vi "Configure PPS.vi"(8 "error in":errorcluster, 11 "PPS Config In":T2={"PPS Operation"=enum."Close", "PowerSupply Instrument"=enum."LVPPS", "Configure"={"Voltage Level (0.0 V)"=0.0, "CURRent Limit (0.0 A)"=0.0, "OVP LEVEL (0V)"=0.0, "OCP LEVEL (0A)"=0.0, "Enable OVP (T: Enable)"=TRUE, "Enable OCP (T: Enable)"=TRUE, "Enable Output "=TRUE, "Delays OCP"=0.0, "Delays OVP"=0.0, "Mode(0:Voltage)"=0, "CURRent Level (0.0 A)"=0.0, "Voltage Limit (0.0 V)"=0.0}} {"Configure"."Voltage Limit (0.0 V)" format="%.2f"; "Configure"."Mode(0:Voltage)" items=["Voltage", "Current"]; "Configure"."OCP LEVEL (0A)" format="%.2f"; "Configure"."OVP LEVEL (0V)" format="%.2f"; "Configure"."Voltage Level (0.0 V)" format="%.2f"}) -> (0 "error out":errorcluster, 3 "PPS Out":T1 {"Actual Current Limit (A)" format="%.2f"; "Actual Voltage Level (V)" format="%.2f"})   [LabVIEW 2023, in "GUI.lvlib" / "Diagnostic.lvlib"]
uses:
  Diagnostic.lvlib
  Control/PPS Configure UI.ctl
  HardwareAbstractionLayer_LVOOP/PowerSupply/Control/PPS Configure Data.ctl
  Control/PPS Out Data UI.ctl
  HardwareAbstractionLayer_LVOOP/PowerSupply/IT-M6018C/IT-M6018C.lvclass
  HardwareAbstractionLayer_LVOOP/PowerSupply/IT-M3904D/IT-M3904D.lvclass
  HardwareAbstractionLayer_LVOOP/PowerSupply/PowerSupply.lvclass
  HardwareAbstractionLayer_LVOOP/Database/Database.lvclass
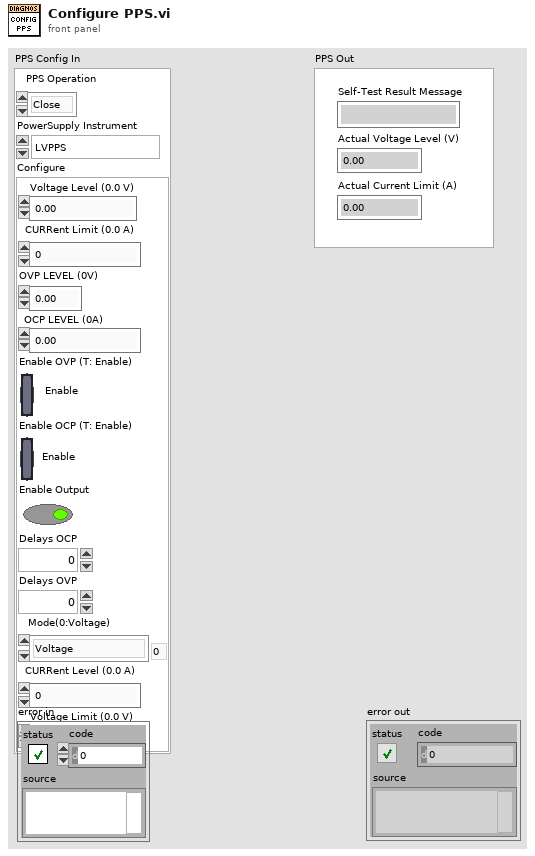
[diagram p1: front panel]
types:
  T1 = typedef "GUI.lvlib/Diagnostic.lvlib/PPS Out Data UI.ctl" = cluster{"Self-Test Result Message":string, "Actual Voltage Level (V)":dbl, "Actual Current Limit (A)":dbl}
  T2 = typedef "GUI.lvlib/Diagnostic.lvlib/PPS Configure UI.ctl" = cluster{"PPS Operation":enum32{"Init", "Self Test", "Configure", "Measure", "Close"}, "PowerSupply Instrument":enum16{"LVPPS", "HVPPS1", "HVPPS2", "HVPPS3", "HVPPS4", "HVPPS5", "HVPPS6"}, "Configure":T3}
  T3 = typedef "HardwareAbstractionLayer_LVOOP.lvlib/PowerSupply.lvclass/PPS Configure Data.ctl" = cluster{"Voltage Level (0.0 V)":dbl, "CURRent Limit (0.0 A)":dbl, "OVP LEVEL (0V)":dbl, "OCP LEVEL (0A)":dbl, "Enable OVP (T: Enable)":bool, "Enable OCP (T: Enable)":bool, "Enable Output ":bool, "Delays OCP":dbl, "Delays OVP":dbl, "Mode(0:Voltage)":u16, "CURRent Level (0.0 A)":dbl, "Voltage Limit (0.0 V)":dbl}
  T4 = enum32{"Init", "Self Test", "Configure", "Measure", "Close"}
  T5 = enum16{"LVPPS", "HVPPS1", "HVPPS2", "HVPPS3", "HVPPS4", "HVPPS5", "HVPPS6"}
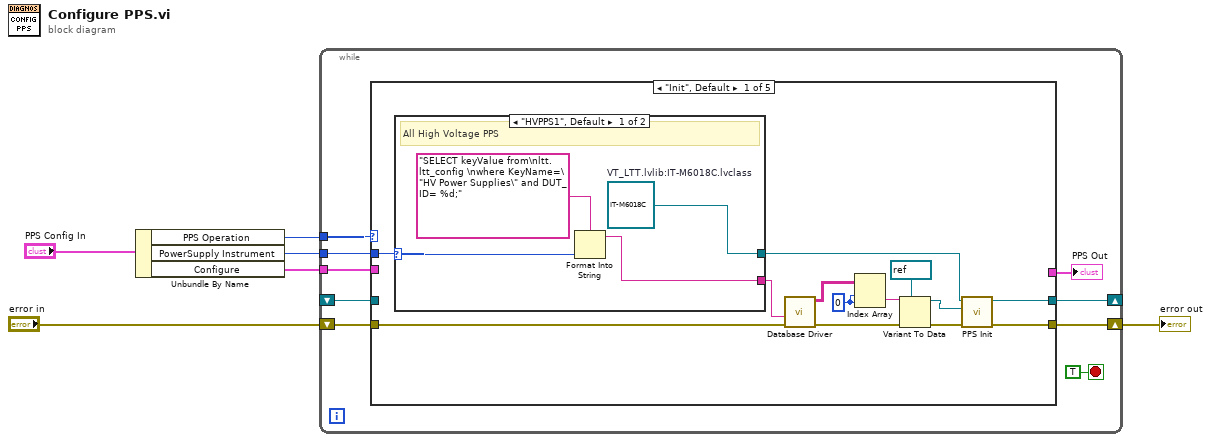
[diagram p0: block diagram]
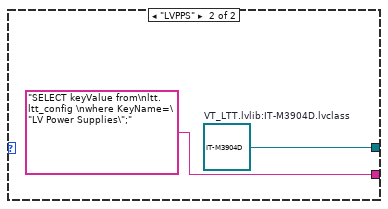
[diagram p2: hidden frame]
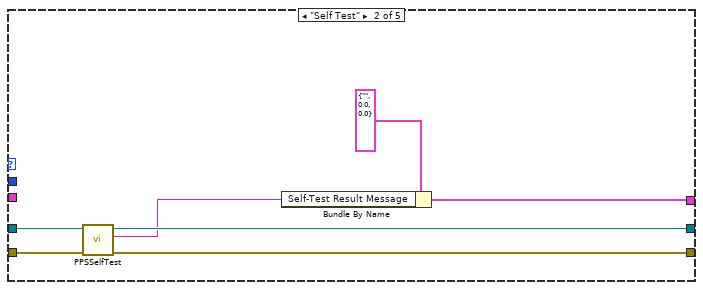
[diagram p3: hidden frame]
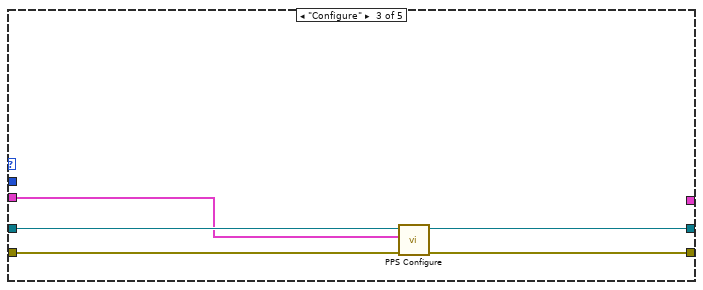
[diagram p4: hidden frame]
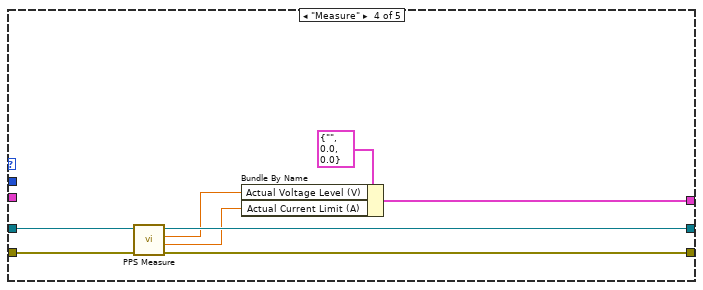
[diagram p5: hidden frame]
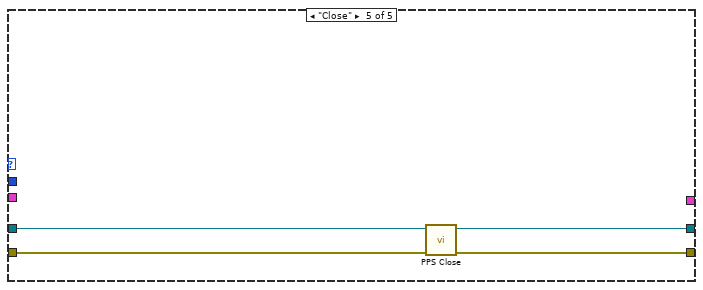
[diagram p6: hidden frame]
diagram:
  n1 = Unbundle By Name("PPS Config In") -> ("PPS Operation"=w6:T4, "PowerSupply Instrument"=w2:T5, "Configure"=w1:T3)
  n2 = while {
    tunnel: w6 -> [w14]
    shift-right: [w11] -> _
    shift-left: _ -> [w10]
    shift-right: [w12] -> w4
    shift-left: "error in" -> [w13]
    tunnel: w2 -> [w8]
    tunnel: w1 -> [w7]
    stop <- TRUE stop-if-true
    n3 = case shown="\"Init\", Default" w14 {
      tunnel: w13 -> [w20 w40 w45 w53 w58]
      tunnel: [w28 w39 w43 w52 w57] -> w12
      tunnel: [w27 w38 w44 w51 w55] -> w11
      tunnel: w10 -> [_ w41 w46 w54 w56]
      tunnel: [_ w35 _ w48 _] -> w9
      tunnel: w8 -> [w16 _ _ _ _]
      tunnel: w7 -> [_ _ w42 _ _]
      frame "Init", Default {
        w26 = 0 ("index (row)")
        n4 = case shown="\"HVPPS1\", Default" w16 {
          selector: w16 -> [w29 _]
          tunnel: [w32 w34] -> w18
          tunnel: [w30 "SELECT keyValue from\nltt.ltt_config \nwhere KeyName=\"LV Power Supplies\";"] -> w22
          frame "HVPPS1", Default {
            w32 = refnum<class "IT-M6018C.lvclass"> refnum  # VT_LTT.lvlib:IT-M6018C.lvclass
            # "All High Voltage PPS"
            n5 = Format Into String(format string="SELECT keyValue from\nltt.ltt_config \nwhere KeyName=\"HV Power Supplies\" and DUT_ID= %d;", w29) -> (resulting string=w30:string)  [unwired: 2 in, 1 out]
          }
          frame "LVPPS" {
            w34 = refnum<class "IT-M3904D.lvclass"> refnum  # VT_LTT.lvlib:IT-M3904D.lvclass
          }
        }
        n6 = call "Database Driver.vi"("error in"=w20, "SQL query"=w22) -> ("error out"=w19:errorcluster, "data"=w21:string[][])  [unwired: 6 in, 2 out]
        n7 = Index Array(array=w21, index (row)=w26, index (col)=w26) -> (element=w23:string)
        n8 = Variant To Data(error in=w19, type=refnum<visa-resource-name> "LV" ("VISA resource name"), Variant=w23) -> (data=w17:refnum<visa-resource-name>, error out=w25:errorcluster)
        n9 = call-dynamic "PPS Init.vi"("error in (no error)"=w25, "VISA resource name"=w17, "PowerSupply in"=w18) -> ("error out"=w28:errorcluster, "PowerSupply out"=w27:refnum<class "PowerSupply.lvclass">)  [unwired: 7 in]
      }
      frame "Self Test" {
        n10 = call-dynamic "PPSSelfTest.vi"("error in (no error)"=w40, "PowerSupply in"=w41) -> ("error out"=w39:errorcluster, "Self-Test Result Message"=w37:string, "PowerSupply out"=w38:refnum<class "PowerSupply.lvclass">)  [unwired: 7 in]
        n11 = Bundle By Name(cluster=T1 {"Self-Test Result Message"="", "Actual Voltage Level (V)"=0.0, "Actual Current Limit (A)"=0.0} ("PPS Out"), "Self-Test Result Message"=w37) -> (w35:T1)
      }
      frame "Configure" {
        n12 = call-dynamic "PPS Configure.vi"("error in (no error)"=w45, "Configure"=w42, "PowerSupply in"=w46) -> ("error out"=w43:errorcluster, "PowerSupply out"=w44:refnum<class "PowerSupply.lvclass">)  [unwired: 7 in]
      }
      frame "Measure" {
        n13 = call-dynamic "PPS Measure.vi"("error in (no error)"=w53, "PowerSupply in"=w54) -> ("error out"=w52:errorcluster, "Actual Current Limit (A)"=w49:dbl, "Actual Voltage Level (V)"=w50:dbl, "PowerSupply out"=w51:refnum<class "PowerSupply.lvclass">)  [unwired: 6 in]
        n14 = Bundle By Name(cluster=T1 {"Self-Test Result Message"="", "Actual Voltage Level (V)"=0.0, "Actual Current Limit (A)"=0.0} ("PPS Out"), "Actual Voltage Level (V)"=w50, "Actual Current Limit (A)"=w49) -> (w48:T1)
      }
      frame "Close" {
        n15 = call-dynamic "PPS Close.vi"("error in (no error)"=w58, "PowerSupply in"=w56) -> ("error out"=w57:errorcluster, "PowerSupply out"=w55:refnum<class "PowerSupply.lvclass">)  [unwired: 8 in]
      }
    }
    "PPS Out" <- w9
  }
  "error out" <- w4
